vi "EXDIR-YAML_IsDashLine.vi"(11 "Line":string) -> (3 "line starts with dash":bool)   [LabVIEW 2016]
panel:
  out "offset of match":i32
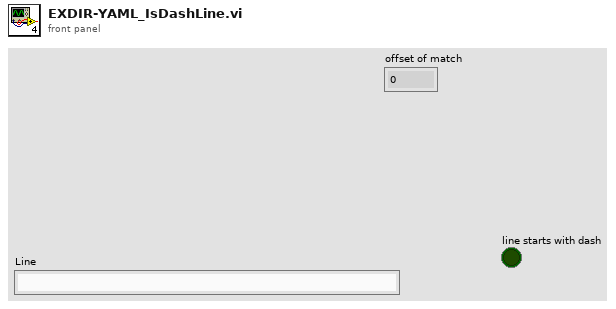
[diagram p1: front panel]
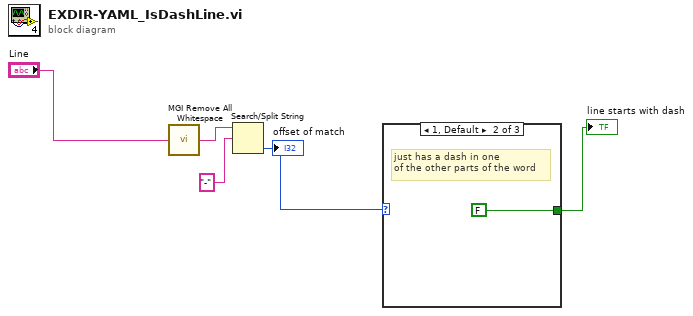
[diagram p0: block diagram]
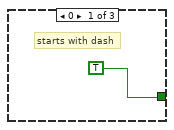
[diagram p2: hidden frame]
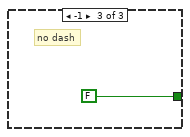
[diagram p3: hidden frame]
diagram:
  n1 = call <userlib>:"MGI Remove All Whitespace.vi"("String"="Line") -> ("Trimmed String"=w4:string)
  n2 = Search/Split String(string=w4, search string/char (-)="-") -> (offset of match=w2:i32)  [unwired: 1 in, 2 out]
  "offset of match" <- w2
  n3 = case shown="1, Default" w2 {
    tunnel: [TRUE FALSE FALSE] -> w1
    frame 0 {
      # "starts with dash"
    }
    frame 1, Default {
      # "just has a dash in one \nof the other parts of the word"
    }
    frame -1 {
      # "no dash"
    }
  }
  "line starts with dash" <- w1
